vi "Update Display.vi"(8 "error in (no error)":errorcluster, 9 "Active Pixels":cluster{"Column":u8, "Row":u8, "Color":u32}[](array[cluster]), 10 "Board State":u32[][](array[numeric]), 11 "Simulated Screen Interface in":refnum<class "Simulated Screen Interface.lvclass">) -> (0 "error out":errorcluster, 3 "Simulated Screen Interface out":refnum<class "Simulated Screen Interface.lvclass">)   [LabVIEW 2017, in "Simulated Screen Interface.lvlib" / "Simulated Screen Interface.lvclass"]
uses:
  Simulated Screen Interface.lvclass
panel:
  out "Board To Display":u32[][](array[numeric])
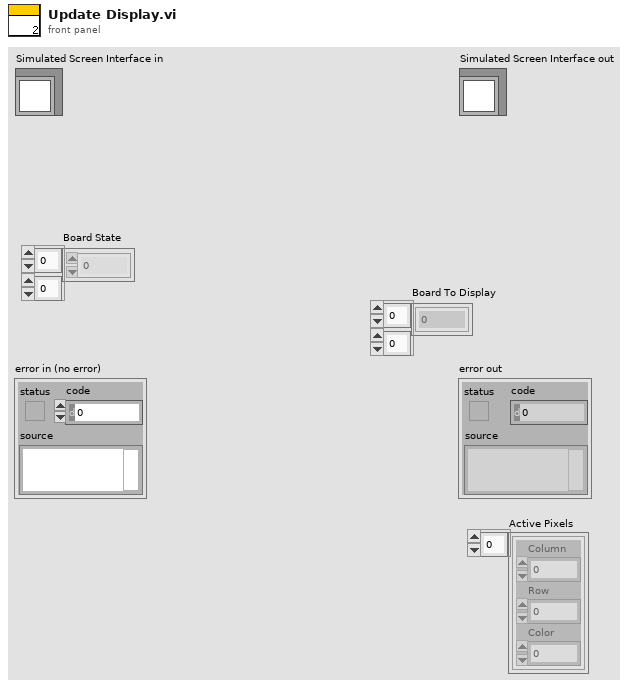
[diagram p1: front panel]
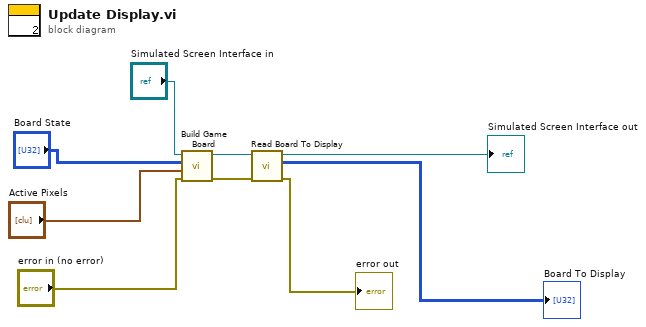
[diagram p0: block diagram]
diagram:
  n1 = call-dynamic "Build Game Board.vi"("error in (no error)"="error in (no error)", "Active Pixels"="Active Pixels", "Board To Draw"="Board State", "Screen Interface in"="Simulated Screen Interface in") -> ("error out"=w3:errorcluster, "Screen Interface out"=w5:refnum<class "Simulated Screen Interface.lvclass">)  [unwired: 6 in]
  n2 = call-dynamic "Read Board To Display.vi"("error in (no error)"=w3, "Screen Interface in"=w5) -> ("error out"=→"error out":errorcluster, "Board To Display"=→"Board To Display":u32[][], "Screen Interface out"=→"Simulated Screen Interface out":refnum<class "Simulated Screen Interface.lvclass">)  [unwired: 7 in]
